vi "DIAction.vi"(6 "Slot":T1, 8 "error in":errorcluster, 11 "CH":string) -> (0 "error out":errorcluster, 3 "Status":bool)   [LabVIEW 2013]
uses:
  SystemCode/SysControl/Slot.ctl
  <vilib>/DAQmx/read.llb/DAQmx Read (Digital Bool 1Line 1Point).vi
  SourceCode/GlobalValue.vi
  <vilib>/DAQmx/create/channels.llb/DAQmx Create Channel (DI-Digital Input).vi
  <vilib>/DAQmx/miscellaneous.llb/DAQmx Fill In Error Info.vi
panel:
  out "lines":tag caption="线"
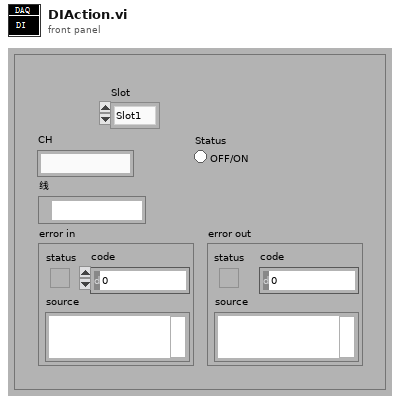
[diagram p1: front panel]
types:
  T1 = typedef "Slot.ctl" = enum16{"Slot1", "Slot2", "Slot3", "Slot4"}
  T2 = typedef "DAQConfig.ctl" = cluster{"DIO":string[][], "AO":string[][], "AI":string[][]}
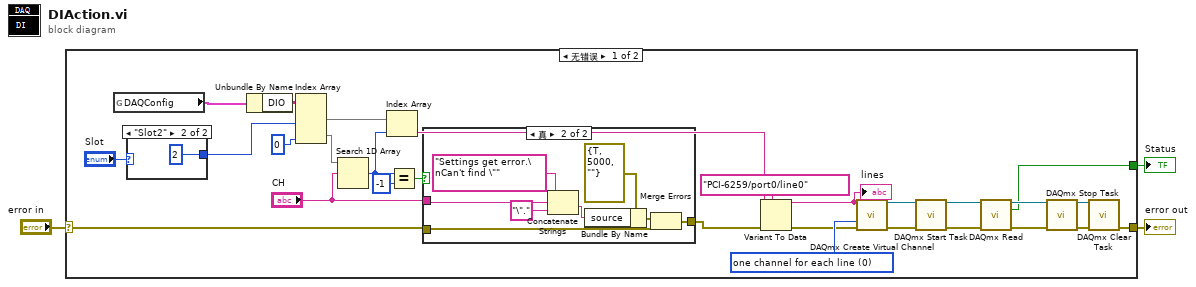
[diagram p0: block diagram]
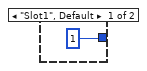
[diagram p2: hidden frame]
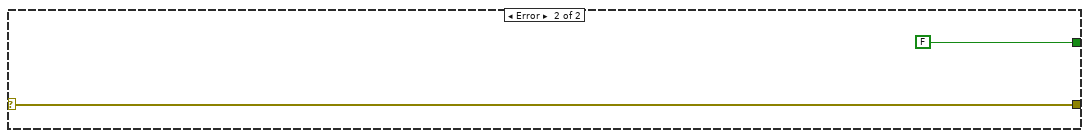
[diagram p4: hidden frame]
diagram:
  n1 = case shown="无错误" "error in" {
    selector: "error in" -> [w10 w44]
    tunnel: [w31 w44] -> w3
    tunnel: [w21 FALSE ("Boolean")] -> w1
    frame No Error {
      w22 = 0 items=["one channel for each line", "one channel for all lines"] ("line grouping")
      n2 = global read "GlobalValue.vi" "DAQConfig"() -> (w4:T2)
      n3 = case shown="\"Slot2\"" "Slot" {
        tunnel: [1 ("索引 (行)") 2 ("索引 (行)")] -> w5
        frame "Slot1", Default {
        }
        frame "Slot2" {
        }
      }
      n4 = Unbundle By Name(w4) -> ("DIO"=w12:string[][])
      n5 = Index Array(array=w12, index (col) #1=w5, index (col) #2=0 ("索引 (列)")) -> (element #1=w7:string[], element #2=w8:string[])  [unwired: 2 in]
      n6 = Search 1D Array(1D array=w8, element="CH") -> (index of element=w14:i32)  [unwired: 1 in]
      n7 = Index Array(array=w7, index=w14) -> (element=w9:string)
      n8 = Equal?(x=w14, y=-1) -> (x = y?=w16:bool)
      n9 = case shown="真" w16 {
        tunnel: "CH" -> [_ w38]
        tunnel: w10 -> [w34 w37]
        tunnel: [w34 w36] -> w11
        frame False {
        }
        frame True {
          n10 = Concatenate Strings("Settings get error.\nCan't find \"" ("message"), w38, "\"." ("string")) -> (w41:string)
          n11 = Bundle By Name(cluster=errorcluster {"status"=TRUE, "code"=5000, "source"=""} ("error in 1 (no error)"), "source"=w41) -> (w40:errorcluster)
          n12 = Merge Errors(w40, w37) -> (w36:errorcluster)
        }
      }
      n13 = Variant To Data(error in=w11, type=tag "PCI-6259/port0/line0" ("lines"), Variant=w9) -> (data=w19:tag, error out=w18:errorcluster)
      "lines" <- w19
      n14 = call-poly <vilib>:"DAQmx Create Virtual Channel.vi"("lines"=w19, "line grouping"=w22, "error in"=w18) -> ("task out"=w30:refnum<k21>, "error out"=w29:errorcluster)  [unwired: 11 in]
      n15 = call <vilib>:"DAQmx Start Task.vi"("task/channels in"=w30, "error in"=w29) -> ("task out"=w28:refnum<k21>, "error out"=w27:errorcluster)  [unwired: 12 in]
      n16 = call-poly <vilib>:"DAQmx Read.vi"("task/channels in"=w28, "error in"=w27) -> ("task out"=w24:refnum<k21>, "data"=w21:bool, "error out"=w23:errorcluster)  [unwired: 11 in]
      n17 = call <vilib>:"DAQmx Stop Task.vi"("task/channels in"=w24, "error in"=w23) -> ("task out"=w26:refnum<k21>, "error out"=w25:errorcluster)  [unwired: 12 in]
      n18 = call <vilib>:"DAQmx Clear Task.vi"("task in"=w26, "error in"=w25) -> ("error out"=w31:errorcluster)  [unwired: 13 in]
    }
    frame Error {
    }
  }
  "error out" <- w3
  "Status" <- w1
